vi "MainStateMachine.vi"(8 "error constant":errorcluster, 11 "FPGA VI Reference In":refnum<k20>) -> (0 "error constant 2":errorcluster, 3 "FPGA VI Reference Out":refnum<k20>)   [LabVIEW 2018]
uses:
  Type_Def/Type_Def ControlState.ctl
  Type_Def/Type_Def ClusterSensor.ctl
  Type_Def/Type_Def Master_DataControl.ctl
  Type_Def/TypeDef_cRIOData.ctl
  Type_Def/Type_Def IMUData.ctl
  Type_Def/TypeDef_BMSData.ctl
  Type_Def/TypeDef_BmsStatus.ctl
  Type_Def/TypeDef FixedMotorData.ctl
  Type_Def/Type_Def Actuator Controls.ctl
  <vilib>/Platform/TimedLoop/XDataNode/timing_clust.ctl
  <vilib>/Platform/TimedLoop/XDataNode/nitl_modes.ctl
  <vilib>/Platform/TimedLoop/XDataNode/wakeup.ctl
  <vilib>/Platform/TimedLoop/XDataNode/loadnilvce.vi
  <vilib>/platform/TimedLoop/XDataNode/XDataNode.xnode
  <vilib>/Platform/TimedLoop/XDataNode/XDNodeRunTimeDep.lvlib
panel:
  in  "SensorData":T1={"cRIO Data"={"HallEffect Right (cm)"=0.0, "HallEffect Left (cm)"=0.0, "Optical Sensor 1 (V)"=0.0, "Optical Sensor 2 (V)"=0.0, "24V Voltage  (V)"=0.0, "24V Current (A)"=0.0, "Contactor H1 Continuity"=0.0, "Contactor L1 Continuity "=0.0, "Contactor H2 Continuity"=0.0, "Contactor L2 Continuity "=0.0, "Brake PT(psig)"=0.0, "Pump PT (psig)"=0.0, "24V Temp   (C)"=0.0, "Tank PT(psig) "=0.0, "ABS Pressure 1 (psig)"=0.0, "ABS Pressure 2 (psig) "=0.0, "Displacement (ft)"=0.0, "Velocity (ft/s)"=0.0, "Time (ms)"=0.0}, "IMU Data"={"x acceleration (g)"=0.0, "Pressure (psia)"=0.0, "Temperature (F)"=0.0}, "BMS Data"={"Pack 1 Max Cell\n Voltage (V)"=0.0, "Pack 1 Max Cell\n ID "=0.0, "Pack 1 Min Cell \nVoltage (V)"=0.0, "Pack 1 Min Cell \nID "=0.0, "Pack 1 State of Charge  (%)"=0.0, "Pack 1 Average Voltage1 (V)"=0.0, "Pack 1Voltage Delta (V)"=0.0, "Pack 1 Current (A)"=0.0, "Pack 1 Voltage (V)"=0.0, "Pack 1 Max Resistance (Ohm)"=0.0, "Pack 1Min Resistance (Ohm)"=0.0, "Pack 1Average Resistance (Ohm)"=0.0, "Pack 1Delta Resistance (Ohm)"=0.0, "Pack 1 Highest Temperature(F)"=0.0, "BmsStatus"={"Pack 1 Fault"=FALSE, "Pack 1 Isolation"=FALSE, "Pack  2 Fault"=FALSE, "Pack 2 Isolation"=FALSE}, "Pack 2 Max Cell\n Voltage (V) "=0.0, "Pack 2 Max Cell\n ID  "=0.0, "Pack 2 Min Cell \nVoltage (V) "=0.0, "Pack 2 Min Cell \nID  "=0.0, "Pack 2 Average Voltage1 (V)"=0.0, "Pack 2 Voltage Delta (V) "=0.0, "Pack 2 Current (A)"=0.0, "Pack 2 Voltage (V) "=0.0, "Pack 2 State of Charge  (%) "=0.0, "Pack 2 Max Resistance (Ohm) "=0.0, "Pack 2 Min Resistance (Ohm)"=0.0, "Pack 2 Average Resistance (Ohm)"=0.0, "Pack 2 Delta Resistance (Ohm) "=0.0, "Pack 2 Highest Temperature(F) "=0.0}, "Motor Data"={" Velocity (RPM)"=0.0, " MotorTemp(C)"=0.0, " ControlTemp(C)"=0.0, " DcLinkVolt(V)"=0.0, " ErrorCode"=0.0, "IsAlive"=FALSE, "motorStatus"={"isReady"=FALSE, "isOn"=FALSE, "isOperEn"=FALSE, "isFault"=FALSE, "isVoltEn"=FALSE, "targetReached"=FALSE, "isWarning"=FALSE}, "motorControllerState"=1}} {"Motor Data"."motorControllerState" items=["unknown"=1, "boot-up"=0, "stopped"=4, "operational"=5, "pre-operational"=127, "connection lost"=128]}
  out "Array":cluster{"SensorCluster":T7}[](array[cluster])
  out "Current State":T8
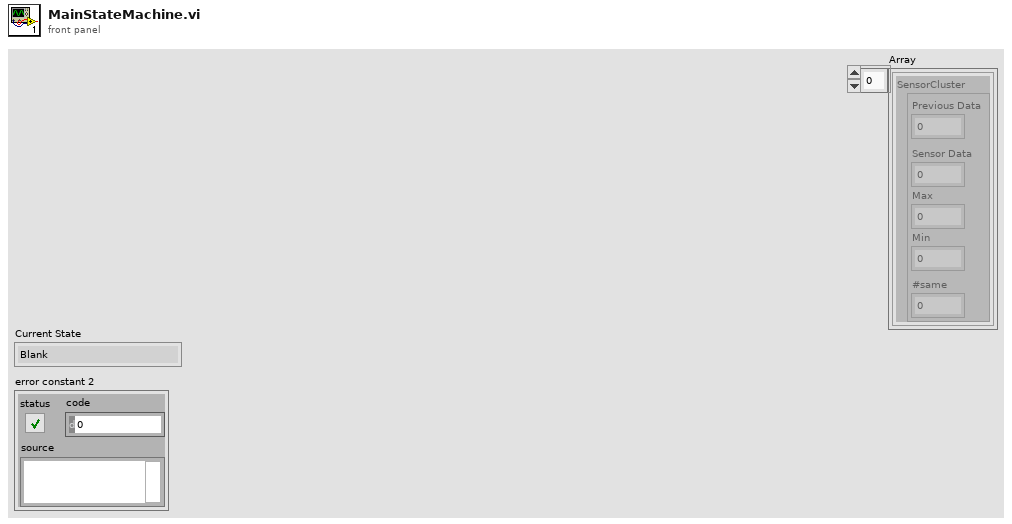
[diagram p1: front panel]
types:
  T1 = typedef "Type_Def Master_DataControl.ctl" = cluster{"cRIO Data":T2, "IMU Data":T3, "BMS Data":T4, "Motor Data":T6}
  T2 = typedef "TypeDef_cRIOData.ctl" = cluster{"HallEffect Right (cm)":dbl, "HallEffect Left (cm)":dbl, "Optical Sensor 1 (V)":dbl, "Optical Sensor 2 (V)":dbl, "24V Voltage  (V)":dbl, "24V Current (A)":dbl, "Contactor H1 Continuity":dbl, "Contactor L1 Continuity ":dbl, "Contactor H2 Continuity":dbl, "Contactor L2 Continuity ":dbl, "Brake PT(psig)":dbl, "Pump PT (psig)":dbl, "24V Temp   (C)":dbl, "Tank PT(psig) ":dbl, "ABS Pressure 1 (psig)":dbl, "ABS Pressure 2 (psig) ":dbl, "Displacement (ft)":dbl, "Velocity (ft/s)":dbl, "Time (ms)":dbl}
  T3 = typedef "Type_Def IMUData.ctl" = cluster{"x acceleration (g)":dbl, "Pressure (psia)":dbl, "Temperature (F)":dbl}
  T4 = typedef "TypeDef_BMSData.ctl" = cluster{"Pack 1 Max Cell\n Voltage (V)":dbl, "Pack 1 Max Cell\n ID ":dbl, "Pack 1 Min Cell \nVoltage (V)":dbl, "Pack 1 Min Cell \nID ":dbl, "Pack 1 State of Charge  (%)":dbl, "Pack 1 Average Voltage1 (V)":dbl, "Pack 1Voltage Delta (V)":dbl, "Pack 1 Current (A)":dbl, "Pack 1 Voltage (V)":dbl, "Pack 1 Max Resistance (Ohm)":dbl, "Pack 1Min Resistance (Ohm)":dbl, "Pack 1Average Resistance (Ohm)":dbl, "Pack 1Delta Resistance (Ohm)":dbl, "Pack 1 Highest Temperature(F)":dbl, "BmsStatus":T5, "Pack 2 Max Cell\n Voltage (V) ":dbl, "Pack 2 Max Cell\n ID  ":dbl, "Pack 2 Min Cell \nVoltage (V) ":dbl, "Pack 2 Min Cell \nID  ":dbl, "Pack 2 Average Voltage1 (V)":dbl, "Pack 2 Voltage Delta (V) ":dbl, "Pack 2 Current (A)":dbl, "Pack 2 Voltage (V) ":dbl, "Pack 2 State of Charge  (%) ":dbl, "Pack 2 Max Resistance (Ohm) ":dbl, "Pack 2 Min Resistance (Ohm)":dbl, "Pack 2 Average Resistance (Ohm)":dbl, "Pack 2 Delta Resistance (Ohm) ":dbl, "Pack 2 Highest Temperature(F) ":dbl}
  T5 = typedef "TypeDef_BmsStatus.ctl" = cluster{"Pack 1 Fault":bool, "Pack 1 Isolation":bool, "Pack  2 Fault":bool, "Pack 2 Isolation":bool}
  T6 = typedef "TypeDef FixedMotorData.ctl" = cluster{" Velocity (RPM)":dbl, " MotorTemp(C)":dbl, " ControlTemp(C)":dbl, " DcLinkVolt(V)":dbl, " ErrorCode":dbl, "IsAlive":bool, "motorStatus":cluster{"isReady":bool, "isOn":bool, "isOperEn":bool, "isFault":bool, "isVoltEn":bool, "targetReached":bool, "isWarning":bool}, "motorControllerState":u16}
  T7 = typedef "Type_Def ClusterSensor.ctl" = cluster{"Sensor Data":dbl, "Max":dbl, "Min":dbl, "Previous Data":dbl, "#same":dbl}
  T8 = typedef "Type_Def ControlState.ctl" = enum16{"Blank", "Systems Check", "Idle", "Ready", "Pushing", "CrawlingPrecharge", "Braking", "Fault", "Boot Up", "Unpowered", "Crawling", "Shutdown", "Service Push", "Service Wait", "Vent", "Precharge"}
  T9 = typedef "Type_Def Actuator Controls.ctl" = cluster{"Reverse ":bool, "Precharge Ctrl":bool, "Pump Ctrl":bool, "24 VDC Ctr":bool, "Vent Solenoid":bool, "Brake Solenoid":bool, "EMCY  Brake Solenoid":bool, "Digital Out 7B ":bool, "Forward Ctrl":bool, "Contact H1":bool, "Contact L1":bool, "Contact H2":bool, "Contact L2 ":bool, "LED RED":bool, "LED GREEN":bool, " Digital Out 7A":bool}
  T10 = typedef "XDNodeRunTimeDep.lvlib/timing_clust.ctl" = cluster{"Expected End [f-1]":u64, "Actual End [f-1]":u64, "Finished Late? [f-1]":bool, "Expected End [i-1]":u64, "Actual End [i-1]":u64, "Finished Late? [i-1]":bool, "Expected Start [i]":u64, "Actual Start [i]":u64, "Expected Start [f]":u64, "Actual Start [f]":u64, "Source Name":string, "Structure Name":string, "Period":i64, "Deadline":i64, "Offset":i64, "Start":i64, "Priority":i32, "Timeout":i32, "Mode":T11, "Wakeup Reason":T12, "Error":errorcluster, "Source Type":string, "Secondary Source Type":string, "Global End Time":u64, "Global Start Time":u64, "Frame Duration":u64, "Iteration Duration":u64, "Assigned CPU":i32, "I/O Scan Engine Mode":u32}
  T11 = typedef "XDNodeRunTimeDep.lvlib/nitl_modes.ctl" = enum32{"No Change", "Process missed periods, maintain original phase", "Discard missed periods, maintain original phase", "Process missed periods, ignore original phase", "Discard missed periods, ignore original phase"}
  T12 = typedef "XDNodeRunTimeDep.lvlib/wakeup.ctl" = enum32{"Normal", "Aborted", "Asynchronous wakeup", "Timing source error", "Timed loop error", "Timeout"}
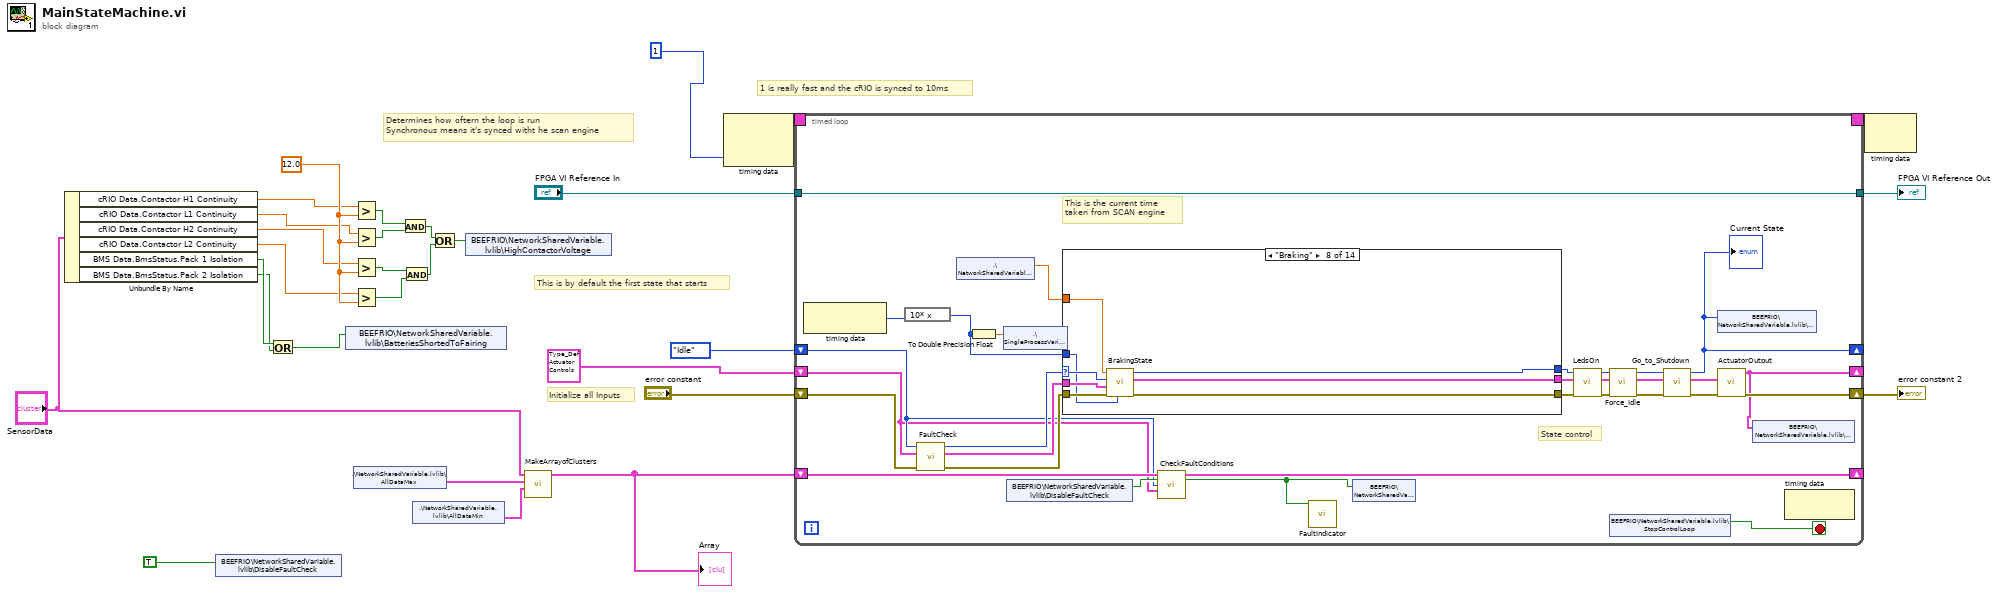
[diagram p0: block diagram]
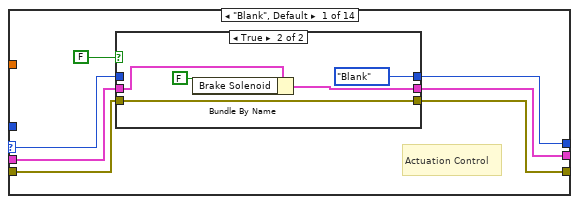
[diagram p2: hidden frame]
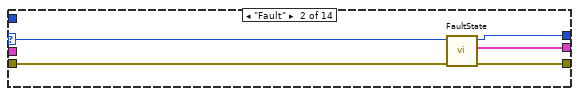
[diagram p4: hidden frame]
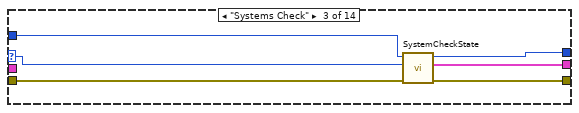
[diagram p5: hidden frame]
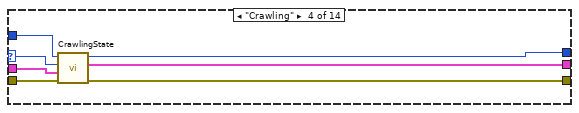
[diagram p6: hidden frame]
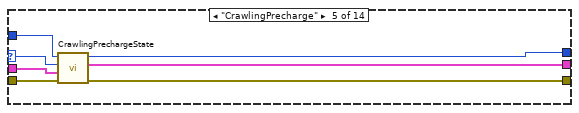
[diagram p7: hidden frame]
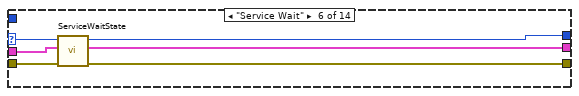
[diagram p8: hidden frame]
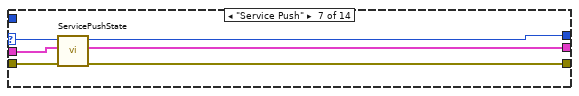
[diagram p9: hidden frame]
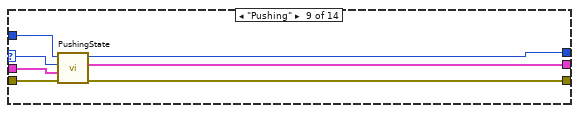
[diagram p10: hidden frame]
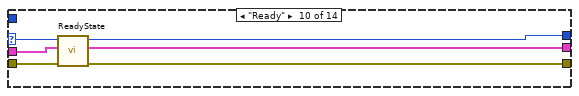
[diagram p11: hidden frame]
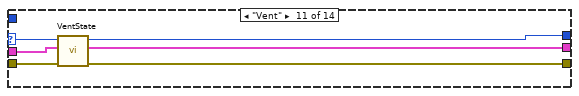
[diagram p12: hidden frame]
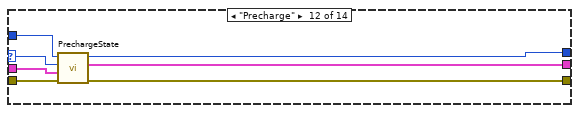
[diagram p13: hidden frame]
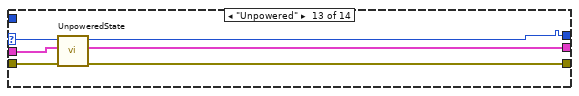
[diagram p14: hidden frame]
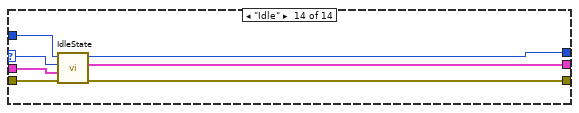
[diagram p15: hidden frame]
diagram:
  w16 = 12.0 ("y")
  # "1 is really fast and the cRIO is synced to 10ms"
  # "Determines how oftern the loop is run \nSynchronous means it's synced witht he scan engine"
  # "Initialize all Inputs"
  # "This is by default the first state that starts"
  n1 = Unbundle By Name("SensorData") -> ("cRIO Data.Contactor H1 Continuity"=w8:dbl, "cRIO Data.Contactor L1 Continuity"=w7:dbl, "cRIO Data.Contactor H2 Continuity"=w6:dbl, "cRIO Data.Contactor L2 Continuity"=w5:dbl, "BMS Data.BmsStatus.Pack 1 Isolation"=w4:bool, "BMS Data.BmsStatus.Pack 2 Isolation"=w3:bool)
  n2 = shared-variable "BEEFRIO\\NetworkSharedVariable.lvlib\\DisableFaultCheck"(TRUE) -> ()  [unwired: 1 in, 1 out]
  n3 = Or(x=w4, y=w3) -> (x .or. y?=w2:bool)
  n4 = shared-variable "BEEFRIO\\NetworkSharedVariable.lvlib\\BatteriesShortedToFairing"(w2) -> ()  [unwired: 1 in, 1 out]
  n5 = Greater?(x=w8, y=w16) -> (0:w15:bool)
  n6 = Greater?(x=w7, y=w16) -> (0:w14:bool)
  n7 = Greater?(x=w6, y=w16) -> (0:w13:bool)
  n8 = Greater?(x=w5, y=w16) -> (0:w1:bool)
  n9 = shared-variable ".\\NetworkSharedVariable.lvlib\\AllDataMax"() -> (w20:T1)  [unwired: 1 in, 1 out]
  n10 = And(x=w15, y=w14) -> (x .and. y?=w12:bool)
  n11 = And(x=w13, y=w1) -> (x .and. y?=w11:bool)
  n12 = shared-variable ".\\NetworkSharedVariable.lvlib\\AllDataMin"() -> (w19:T1)  [unwired: 1 in, 1 out]
  n13 = Or(x=w12, y=w11) -> (x .or. y?=w10:bool)
  n14 = shared-variable "BEEFRIO\\NetworkSharedVariable.lvlib\\HighContactorVoltage"(w10) -> ()  [unwired: 1 in, 1 out]
  n15 = call "MakeArrayofClusters.vi"("AllDataMin"=w19, "AllDataMax"=w20, "SensorData"="SensorData") -> ("Array"=w24:cluster{"SensorCluster":T7}[])  [unwired: 8 in]
  "Array" <- w24
  n16 = node-c288 ("Input Node")(i64 1 ("Period")) -> (w29:T10)  [unwired: 1 in]
  n17 = timed-loop "Timed Loop" {
    timing: w29 -> [_]
    timing-out: [_] -> w28
    shift-right: [w39] -> _
    shift-left: Type_Def_ControlState."Idle" -> [w46]
    shift-right: [w34] -> _
    shift-left: T9 {"Reverse "=FALSE, "Precharge Ctrl"=FALSE, "Pump Ctrl"=FALSE, "24 VDC Ctr"=FALSE, "Vent Solenoid"=FALSE, "Brake Solenoid"=FALSE, "EMCY  Brake Solenoid"=FALSE, "Digital Out 7B "=FALSE, "Forward Ctrl"=FALSE, "Contact H1"=FALSE, "Contact L1"=FALSE, "Contact H2"=FALSE, "Contact L2 "=FALSE, "LED RED"=FALSE, "LED GREEN"=FALSE, " Digital Out 7A"=FALSE} -> [w45]
    shift-right: [w54] -> w21
    shift-left: "error constant" -> [w59]
    shift-right: [w49] -> _
    shift-left: w24 -> [w48]
    tunnel: [w43] -> w23
    tunnel: "FPGA VI Reference In" -> [w43]
    stop <- w44 stop-if-true
    # "State control"
    # "This is the current time \ntaken from SCAN engine"
    n18 = node-c288() -> (w56:i64)  [unwired: 1 in]
    n19 = expression code="10* x"(w56) -> (w55:i64)
    n20 = call "FaultCheck.vi"("error in (no error)"=w59, "Cluster in"=w45, "Enum in"=w46) -> ("error out"=w50:errorcluster, "Cluster out"=w51:T9, "Enum out"=w52:T8)  [unwired: 6 in]
    n21 = shared-variable ".\\NetworkSharedVariable.lvlib\\Velocity"() -> (w53:dbl)  [unwired: 1 in, 1 out]
    n22 = To Double Precision Float(number=w55) -> (double precision float=w35:dbl)
    n23 = shared-variable ".\\SingleProcessVariable.lvlib\\Time"(w35) -> ()  [unwired: 1 in, 1 out]
    n24 = shared-variable "BEEFRIO\\NetworkSharedVariable.lvlib\\DisableFaultCheck"() -> (w47:bool)  [unwired: 1 in, 1 out]
    n25 = case shown="\"Braking\"" w52 {
      selector: w52 -> [w66 w76 w81 w92 w99 w105 w111 w119 w126 w132 w138 w145 w151 w158]
      tunnel: [w64 w77 w82 w90 w97 w103 w109 w117 w124 w130 w136 w143 w149 w156] -> w58
      tunnel: w51 -> [w65 _ _ w91 w98 w104 w110 w118 w125 w131 w137 w144 w150 w157]
      tunnel: [w63 w78 w83 w89 w96 w102 w108 w116 w123 w129 w135 w142 w148 w155] -> w57
      tunnel: w50 -> [w62 w79 w84 w88 w95 w101 w107 w115 w122 w128 w134 w141 w147 w154]
      tunnel: w55 -> [_ _ w85 w87 w94 _ _ w112 w121 _ _ w140 _ w153]
      tunnel: w53 -> [_ _ _ _ _ _ _ w114 _ _ _ _ _ _]
      tunnel: [w60 w75 w80 w86 w93 w100 w106 w113 w120 w127 w133 w139 w146 w152] -> w36
      frame "Blank", Default {
        # "Actuation Control"
        n26 = case shown="True" FALSE {
          tunnel: w66 -> [w69 _]
          tunnel: [w69 Type_Def_ControlState."Blank"] -> w60
          tunnel: w65 -> [w68 w73]
          tunnel: [w68 w71] -> w64
          tunnel: [w67 w70] -> w63
          tunnel: w62 -> [w67 w70]
          frame False {
          }
          frame True {
            n27 = Bundle By Name(cluster=w73, "Brake Solenoid"=FALSE ("Digital Out 5")) -> (w71:T9)
          }
        }
      }
      frame "Fault" {
        n28 = call "FaultState.vi"("error in (no error)"=w79, "CurrentState"=w76) -> ("error out"=w78:errorcluster, "Cluster"=w77:T9, "CurrentState 2"=w75:T8)  [unwired: 7 in]
      }
      frame "Systems Check" {
        n29 = call "SystemCheckState.vi"("error in (no error)"=w84, "State in"=w81, "Actual Start [i]"=w85) -> ("error out"=w83:errorcluster, "Cluster"=w82:T9, "State Out"=w80:T8)  [unwired: 5 in]
      }
      frame "Crawling" {
        n30 = call "CrawlingState.vi"("error in (no error)"=w88, "Cluster in"=w91, "Enum in"=w92, "Actual Start [i]"=w87) -> ("error out"=w89:errorcluster, "Cluster out"=w90:T9, "Enum"=w86:T8)  [unwired: 5 in]
      }
      frame "CrawlingPrecharge" {
        n31 = call "CrawlingPrechargeState.vi"("error in (no error)"=w95, "Cluster in"=w98, "Enum in"=w99, "Actual Start [i]"=w94) -> ("error out"=w96:errorcluster, "Cluster out"=w97:T9, "Enum"=w93:T8)  [unwired: 5 in]
      }
      frame "Service Wait" {
        n32 = call "ServiceWaitState.vi"("error in (no error)"=w101, "Cluster in"=w104, "Enum in"=w105) -> ("error out"=w102:errorcluster, "Cluster out"=w103:T9, "Enum"=w100:T8)  [unwired: 6 in]
      }
      frame "Service Push" {
        n33 = call "ServicePushState.vi"("error in (no error)"=w107, "Cluster in"=w110, "Enum in"=w111) -> ("error out"=w108:errorcluster, "Cluster out"=w109:T9, "Enum out"=w106:T8)  [unwired: 6 in]
      }
      frame "Braking" {
        n34 = call "BrakingState.vi"("Actual Start [i]"=w112, "error in (no error)"=w115, "Cluster in"=w118, "Enum in"=w119, "Velocity"=w114) -> ("error out"=w116:errorcluster, "Cluster"=w117:T9, "Enum"=w113:T8)  [unwired: 4 in]
      }
      frame "Pushing" {
        n35 = call "PushingState.vi"("error in (no error)"=w122, "Cluster in"=w125, "Enum in"=w126, "Actual Start [i]"=w121) -> ("error out"=w123:errorcluster, "Cluster out"=w124:T9, "Enum"=w120:T8)  [unwired: 5 in]
      }
      frame "Ready" {
        n36 = call "ReadyState.vi"("error in (no error)"=w128, "Cluster in"=w131, "Enum in"=w132) -> ("error out"=w129:errorcluster, "Cluster out"=w130:T9, "Enum"=w127:T8)  [unwired: 6 in]
      }
      frame "Vent" {
        n37 = call "VentState.vi"("error in (no error)"=w134, "Cluster in"=w137, "Enum in"=w138) -> ("error out"=w135:errorcluster, "Cluster out"=w136:T9, "Enum out"=w133:T8)  [unwired: 6 in]
      }
      frame "Precharge" {
        n38 = call "PrechargeState.vi"("error in (no error)"=w141, "Cluster in"=w144, "Enum in"=w145, "Actual Start [i]"=w140) -> ("error out"=w142:errorcluster, "Cluster out"=w143:T9, "Enum"=w139:T8)  [unwired: 5 in]
      }
      frame "Unpowered" {
        n39 = call "UnpoweredState.vi"("error in (no error)"=w147, "Cluster in"=w150, "Enum in"=w151) -> ("error out"=w148:errorcluster, "Cluster out"=w149:T9, "Enum"=w146:T8)  [unwired: 6 in]
      }
      frame "Idle" {
        n40 = call "IdleState.vi"("error in (no error)"=w154, "Cluster in"=w157, "Enum in"=w158, "Actual Start [i]"=w153) -> ("error out"=w155:errorcluster, "Cluster out"=w156:T9, "Enum"=w152:T8)  [unwired: 5 in]
      }
    }
    n41 = call "CheckFaultConditions.vi"("Array 2"=w48, "DisableFaultCheck"=w47, "ControlState"=w46, 9:w45) -> ("Array out"=w49:cluster{"SensorCluster":T7}[], "Fault?"=w33:bool)  [unwired: 10 in]
    n42 = call "FaultIndicator.vi"("Fault in"=w33) -> ()  [unwired: 11 in]
    n43 = shared-variable "BEEFRIO\\NetworkSharedVariable.lvlib\\Fault"(w33) -> ()  [unwired: 1 in, 1 out]
    n44 = call "LedsOn"("error in (no error)"=w57, "Cluster in"=w58, "Enum in"=w36) -> ("error out"=w31:errorcluster, "Cluster"=w32:T9, "Enum out"=w30:T8)  [unwired: 6 in]
    n45 = call "Force_Idle.vi"("error in (no error)"=w31, "Cluster in"=w32, "Enum in"=w30) -> ("error out"=w38:errorcluster, "Cluster out"=w42:T9, "Enum out"=w40:T8)  [unwired: 6 in]
    n46 = shared-variable "BEEFRIO\\NetworkSharedVariable.lvlib\\StopControlLoop"() -> (w44:bool)  [unwired: 1 in, 1 out]
    n47 = call "Go_to_Shutdown.vi"("error in (no error)"=w38, "Cluster in"=w42, "Enum in"=w40) -> ("error out"=w37:errorcluster, "Cluster out"=w41:T9, "Enum out"=w39:T8)  [unwired: 5 in, 1 out]
    "Current State" <- w39
    n48 = shared-variable "BEEFRIO\\NetworkSharedVariable.lvlib\\CurrentState"(w39) -> ()  [unwired: 1 in, 1 out]
    n49 = call "ActuatorOutput.vi"("error in (no error)"=w37, "Cluster in"=w41) -> ("error out"=w54:errorcluster, "Cluster"=w34:T9)  [unwired: 8 in]
    n50 = shared-variable "BEEFRIO\\NetworkSharedVariable.lvlib\\ActuationList"(w34) -> ()  [unwired: 1 in, 1 out]
    n51 = node-c288() -> ()  [unwired: 1 in, 1 out]
  }
  "FPGA VI Reference Out" <- w23
  "error constant 2" <- w21
  n52 = node-c288(w28) -> ()  [unwired: 1 out]
